vi "toggle.vi"(1 "Input":bool) -> (0 "Output/Shift Register":bool)   [LabVIEW 2011]
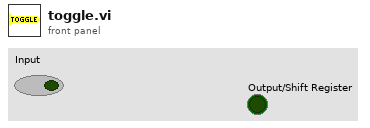
[diagram p1: front panel]
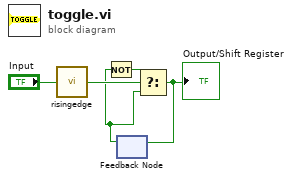
[diagram p0: block diagram]
diagram:
  n1 = call "risingedge.vi"("Input"="Input") -> ("Output"=w4:bool)
  n2 = feedback #1() -> (w1:bool)  [unwired: 1 in]
  n3 = Not(x=w1) -> (.not. x?=w3:bool)
  n4 = Select(t=w3, s=w4, f=w1) -> (s? t:f=w2:bool)
  "Output/Shift Register" <- w2
  n5 = feedback-in #1(w2) -> ()
